vi "Freefield-Default Arguments.vi"() -> (4 "Folder out":path, 6 "Endpoints out":T1[](array[typedef]), 8 "Mic device out":string, 15 "error out":errorcluster)   [LabVIEW 2020]
uses:
  Common VIs/Typedefs/CAL-Endpoint.ctl
  <vilib>/Utility/sysdir.llb/System Directory Type.ctl
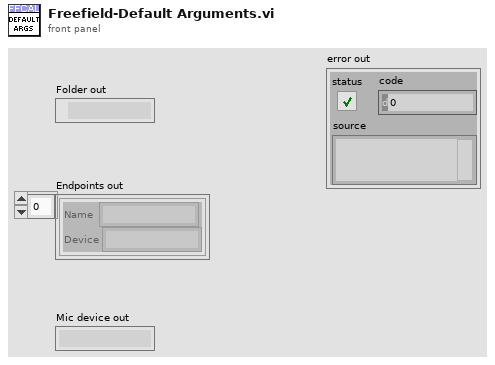
[diagram p1: front panel]
types:
  T1 = typedef "CAL-Endpoint.ctl" = cluster{"Name":string, "Device":string}
  T2 = typedef "System Directory Type.ctl" = i32
  T3 = typedef "TDT-Output source.ctl" = cluster{"Device":T4, "Num":i32}
  T4 = typedef "TDT-Device ID.ctl" = enum16{"None", "PA5", "RP2", "RL2", "RA16", "RV8", "RX5", "RX6", "RX7", "RX8", "RZ2", "RZ5", "RZ6"}
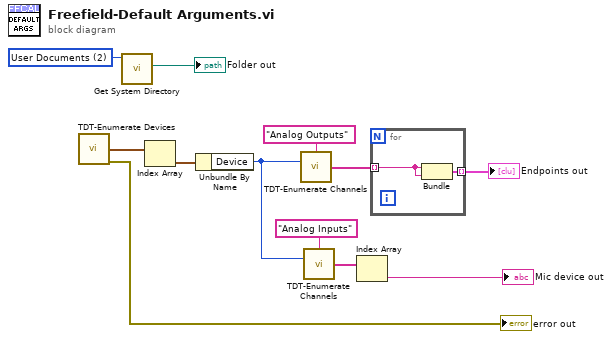
[diagram p0: block diagram]
diagram:
  w12 = T2 2 items=["User Home"=0, "User Desktop"=1, "User Documents"=2, "User Application Data"=3, "User Preferences"=4, "User Temporary"=5, "Public Documents"=6, "Public Application Data"=7, "Public Preferences"=8, "Public Cache"=13, "System Core Libraries"=9, "System Installed Libraries"=10, "Application Files"=11, "Boot Volume Root"=12] ("system directory type")
  n1 = call "TDT-Enumerate Devices.vi"() -> ("Devices"=w10:T3[], "error out"=→"error out":errorcluster)  [unwired: 14 in]
  n2 = call <vilib>:"Get System Directory.vi"("system directory type"=w12) -> ("system directory"=→"Folder out":path)  [unwired: 10 in]
  n3 = Index Array(array=w10) -> (element=w9:T3)  [unwired: 1 in]
  n4 = Unbundle By Name(w9) -> ("Device"=w4:T4)
  n5 = call "TDT-Enumerate Channels.vi"("Type"="Analog Outputs", "IO Device"=w4) -> ("IO Channels"=w7:string[])  [unwired: 13 in]
  n6 = call "TDT-Enumerate Channels.vi"("Type"="Analog Inputs", "IO Device"=w4) -> ("IO Channels"=w3:string[])  [unwired: 13 in]
  n7 = Index Array(array=w3) -> (element=→"Mic device out":string)  [unwired: 1 in]
  n8 = for {
    tunnel: w7 -> [w14] mode=indexing
    tunnel: [w13] -> w6 mode=indexing
    n9 = Bundle(w14, w14) -> (w13:cluster{string, string})  [unwired: 1 in]
  }
  "Endpoints out" <- w6
